vi "bt_test1.vi"() -> ()   [LabVIEW 2025]
panel:
  in  "Python interpreter Path":path
  out "error out":errorcluster
  in  "b":dbl
  in  "a":dbl
  out "a+b":dbl
  in  "Python Script Path":path
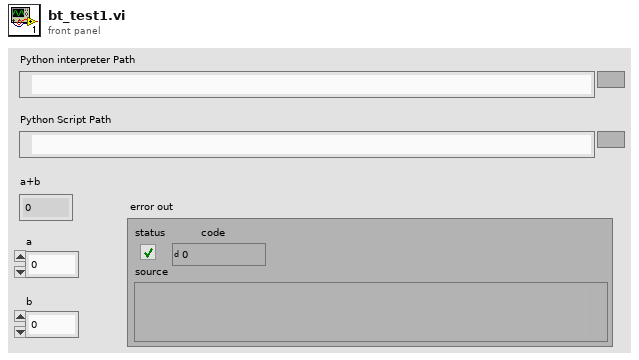
[diagram p1: front panel]
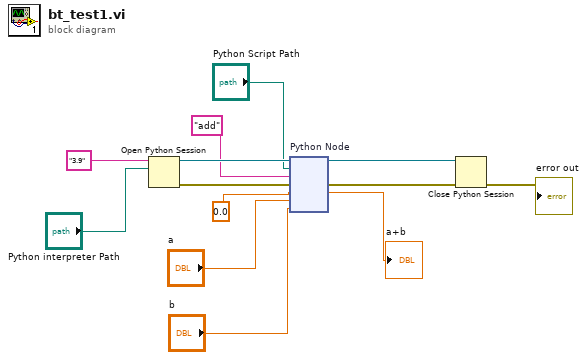
[diagram p0: block diagram]
diagram:
  n1 = Open Python Session(python version="3.9", python path="Python interpreter Path") -> (session out=w13:refnum<k35>, error out=w8:errorcluster)  [unwired: 1 in]
  n2 = node "Python Node"(w13, "Python Script Path", "add", w8, 0.0, "a", "b") -> (w12:refnum<k35>, w7:errorcluster, →"a+b":dbl)  [unwired: 2 in, 2 out]
  n3 = Close Python Session(session in=w12, error in=w7) -> (11:→"error out":errorcluster)
